vi "Open Section Datas.vi"(8 "error in (no error)":errorcluster, 11 "Data in":string) -> (0 "error out":errorcluster, 3 "Section":refnum<data-value>)   [LabVIEW 2013, in "Hierarchy Framework.lvlib" / "Section.lvclass"]
uses:
  Section.lvclass
  Channel/Channel.lvclass
  Channel/Ctls/Dimensions.ctl
  Item/Item.lvclass
  Generic/Generic.lvclass
panel:
  out "String":string
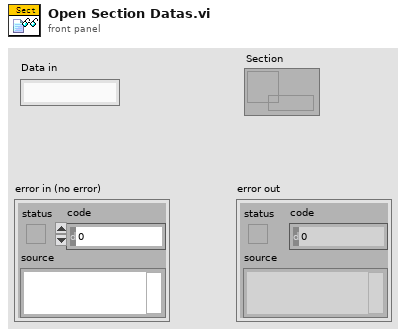
[diagram p1: front panel]
types:
  T1 = typedef "Hierarchy Framework.lvlib/Channel.lvclass/Dimensions.ctl" = cluster{"Row":i32, "Column":i32}
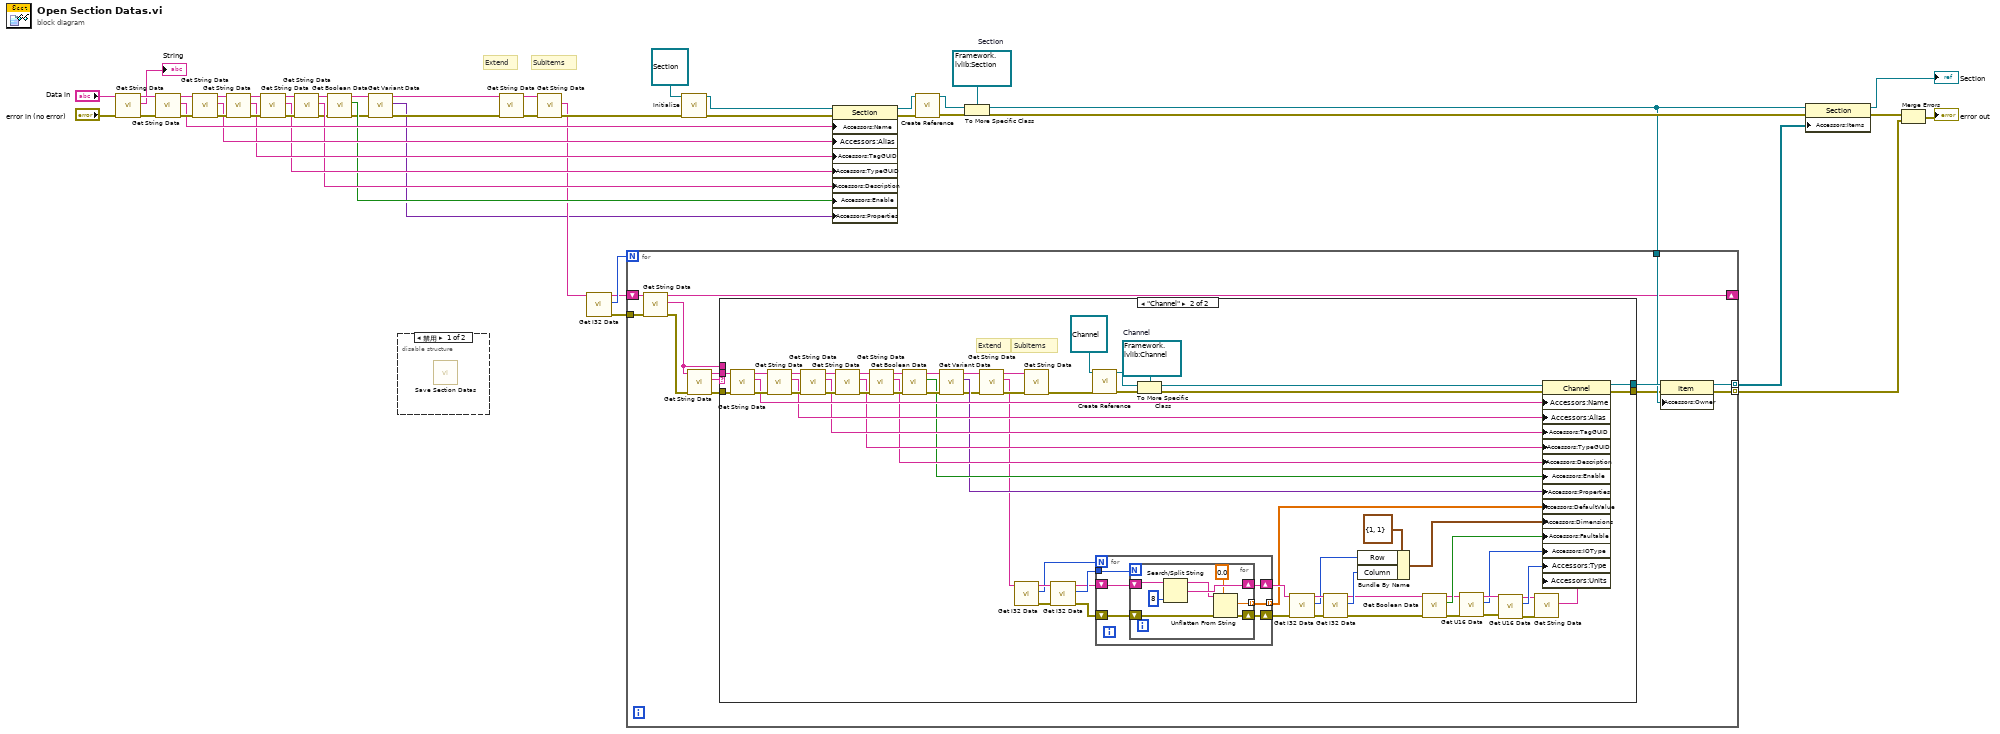
[diagram p0: block diagram]
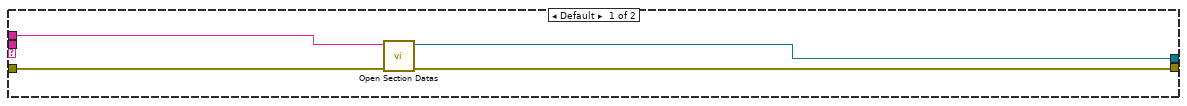
[diagram p2: hidden frame]
diagram:
  w45 = refnum<data-value> refnum  # Section
  # "SubItems"
  # "Extend"
  n1 = call "Get String Data.vi"("error in (no error)"="error in (no error)", "Data in"="Data in") -> ("error out"=w33:errorcluster, "String"=→"String":string, "Data out"=w34:string)  [unwired: 7 in]
  n2 = call "Get String Data.vi"("error in (no error)"=w33, "Data in"=w34) -> ("error out"=w26:errorcluster, "String"=w24:string, "Data out"=w28:string)  [unwired: 7 in]
  n3 = call "Get String Data.vi"("error in (no error)"=w26, "Data in"=w28) -> ("error out"=w32:errorcluster, "String"=w23:string, "Data out"=w31:string)  [unwired: 7 in]
  n4 = call "Get String Data.vi"("error in (no error)"=w32, "Data in"=w31) -> ("error out"=w25:errorcluster, "String"=w22:string, "Data out"=w27:string)  [unwired: 7 in]
  n5 = call "Get String Data.vi"("error in (no error)"=w25, "Data in"=w27) -> ("error out"=w29:errorcluster, "String"=w21:string, "Data out"=w30:string)  [unwired: 7 in]
  n6 = call "Get String Data.vi"("error in (no error)"=w29, "Data in"=w30) -> ("error out"=w17:errorcluster, "String"=w20:string, "Data out"=w18:string)  [unwired: 7 in]
  n7 = call "Get Boolean Data.vi"("error in (no error)"=w17, "Data in"=w18) -> ("error out"=w7:errorcluster, "Boolean"=w16:bool, "Data out"=w8:string)  [unwired: 7 in]
  n8 = call "Get Variant Data.vi"("error in (no error)"=w7, "Data in"=w8) -> ("error out"=w5:errorcluster, "Variant"=w4:variant, "Data out"=w6:string)  [unwired: 7 in]
  n9 = disable-structure shown="禁用" {
    frame Disabled {
      n10 = call "Save Section Datas.vi"() -> ()  [unwired: 9 in, 3 out]
    }
    frame Enabled {
    }
  }
  n11 = call "Get String Data.vi"("error in (no error)"=w5, "Data in"=w6) -> ("error out"=w15:errorcluster, "Data out"=w14:string)  [unwired: 7 in, 1 out]
  n12 = call "Get String Data.vi"("error in (no error)"=w15, "Data in"=w14) -> ("error out"=w13:errorcluster, "String"=w9:string)  [unwired: 7 in, 1 out]
  n13 = call "Get I32 Data.vi"("Data in"=w9) -> ("error out"=w10:errorcluster, "I32"=w12:i32, "Data out"=w11:string)  [unwired: 8 in]
  n14 = call-dynamic "Initialize.vi"("error in (no error)"=w13, "Section输入"=refnum<class "Section.lvclass"> refnum ("Framework.lvlib:Section")) -> ("error out"=w39:errorcluster, "Section输出"=w38:refnum<class "Section.lvclass">)  [unwired: 8 in]
  n15 = property class="Section"(reference=w38, error in=w39, "Accessors:Name"=w24, "Accessors:Alias"=w23, "Accessors:TagGUID"=w22, "Accessors:TypeGUID"=w21, "Accessors:Description"=w20, "Accessors:Enable"=w16, "Accessors:Properties"=w4) -> (reference out=w41:refnum<class "Section.lvclass">, error out=w42:errorcluster)
  n16 = call "Create Reference.vi"("error in (no error)"=w42, "Generic"=w41) -> ("error out"=w44:errorcluster, "Generic Reference"=w43:refnum<data-value>)  [unwired: 8 in]
  n17 = To More Specific Class(target class=w45, reference=w43, error in=w44) -> (specific class reference=w37:refnum<data-value>, error out=w46:errorcluster)
  n18 = for {
    N: w12 -> [_]
    tunnel: [w60] -> w47 mode=indexing
    tunnel: w37 -> [w59]
    shift-right: [w57] -> _
    shift-left: w11 -> [w58]
    tunnel: w10 -> [w56]
    tunnel: [w49] -> w2 mode=indexing
    n19 = call "Get String Data.vi"("error in (no error)"=w56, "Data in"=w58) -> ("error out"=w51:errorcluster, "String"=w52:string, "Data out"=w57:string)  [unwired: 7 in]
    n20 = call "Get String Data.vi"("error in (no error)"=w51, "Data in"=w52) -> ("error out"=w53:errorcluster, "String"=w55:string, "Data out"=w54:string)  [unwired: 7 in]
    n21 = case shown="\"Channel\"" w55 {
      tunnel: [w65 w121] -> w61
      tunnel: w54 -> [_ w112]
      tunnel: w53 -> [w63 w111]
      tunnel: w52 -> [w64 _]
      tunnel: [w62 w66] -> w50
      frame Default {
        n22 = call "Open Section Datas.vi"("error in (no error)"=w63, "Data in"=w64) -> ("error out"=w62:errorcluster, "Section"=w65:refnum<data-value>)  [unwired: 8 in]
      }
      frame "Channel" {
        w124 = refnum<data-value> refnum  # Channel
        # "SubItems"
        # "Extend"
        n23 = call "Get String Data.vi"("error in (no error)"=w111, "Data in"=w112) -> ("error out"=w110:errorcluster, "String"=w104:string, "Data out"=w118:string)  [unwired: 7 in]
        n24 = call "Get String Data.vi"("error in (no error)"=w110, "Data in"=w118) -> ("error out"=w109:errorcluster, "String"=w103:string, "Data out"=w120:string)  [unwired: 7 in]
        n25 = call "Get String Data.vi"("error in (no error)"=w109, "Data in"=w120) -> ("error out"=w108:errorcluster, "String"=w102:string, "Data out"=w117:string)  [unwired: 7 in]
        n26 = call "Get String Data.vi"("error in (no error)"=w108, "Data in"=w117) -> ("error out"=w107:errorcluster, "String"=w101:string, "Data out"=w119:string)  [unwired: 7 in]
        n27 = call "Get String Data.vi"("error in (no error)"=w107, "Data in"=w119) -> ("error out"=w106:errorcluster, "String"=w100:string, "Data out"=w116:string)  [unwired: 7 in]
        n28 = call "Get Boolean Data.vi"("error in (no error)"=w106, "Data in"=w116) -> ("error out"=w105:errorcluster, "Boolean"=w99:bool, "Data out"=w115:string)  [unwired: 7 in]
        n29 = call "Get Variant Data.vi"("error in (no error)"=w105, "Data in"=w115) -> ("error out"=w67:errorcluster, "Variant"=w98:variant, "Data out"=w114:string)  [unwired: 7 in]
        n30 = call "Get String Data.vi"("error in (no error)"=w67, "Data in"=w114) -> ("error out"=w97:errorcluster, "String"=w95:string, "Data out"=w113:string)  [unwired: 7 in]
        n31 = call "Get I32 Data.vi"("Data in"=w95) -> ("error out"=w93:errorcluster, "I32"=w92:i32, "Data out"=w94:string)  [unwired: 8 in]
        n32 = call "Get String Data.vi"("error in (no error)"=w97, "Data in"=w113) -> ("error out"=w96:errorcluster)  [unwired: 7 in, 2 out]
        n33 = call "Get I32 Data.vi"("error in (no error)"=w93, "Data in"=w94) -> ("error out"=w89:errorcluster, "I32"=w91:i32, "Data out"=w90:string)  [unwired: 7 in]
        n34 = call "Create Reference.vi"("error in (no error)"=w96, "Generic"=refnum<class "Channel.lvclass"> refnum ("Framework.lvlib:Channel")) -> ("error out"=w125:errorcluster, "Generic Reference"=w126:refnum<data-value>)  [unwired: 8 in]
        n35 = for {
          N: w92 -> [_]
          shift-right: [w131] -> w86
          shift-left: w90 -> [w132]
          tunnel: w91 -> [w133]
          tunnel: [w130] -> w85 mode=indexing
          shift-right: [w128] -> w84
          shift-left: w89 -> [w129]
          n36 = for {
            N: w133 -> [_]
            shift-right: [w139] -> w131
            shift-left: w132 -> [w141]
            tunnel: [w136] -> w130 mode=indexing
            shift-right: [w134] -> w128
            shift-left: w129 -> [w135]
            n37 = Search/Split String(string=w141, offset (0)=8 ("偏移量(0)")) -> (substring before match=w138:string, match + rest of string=w139:string)  [unwired: 1 in, 1 out]
            n38 = Unflatten From String(type=0.0 ("数值"), binary string=w138, error in (no error)=w135) -> (value=w136:dbl, error out=w134:errorcluster)  [unwired: 2 in, 1 out]
          }
        }
        n39 = To More Specific Class(target class=w124, reference=w126, error in=w125) -> (specific class reference=w123:refnum<data-value>, error out=w122:errorcluster)
        n40 = call "Get I32 Data.vi"("error in (no error)"=w84, "Data in"=w86) -> ("error out"=w88:errorcluster, "I32"=w81:i32, "Data out"=w87:string)  [unwired: 7 in]
        n41 = call "Get I32 Data.vi"("error in (no error)"=w88, "Data in"=w87) -> ("error out"=w78:errorcluster, "I32"=w80:i32, "Data out"=w79:string)  [unwired: 7 in]
        n42 = Bundle By Name(cluster=T1 {"Row"=1, "Column"=1} ("Dimensions"), "Row"=w81, "Column"=w80) -> (w82:T1)
        n43 = call "Get Boolean Data.vi"("error in (no error)"=w78, "Data in"=w79) -> ("error out"=w73:errorcluster, "Boolean"=w77:bool, "Data out"=w74:string)  [unwired: 7 in]
        n44 = call "Get U16 Data.vi"("error in (no error)"=w73, "Data in"=w74) -> ("error out"=w76:errorcluster, "U16"=w72:u16, "Data out"=w75:string)  [unwired: 7 in]
        n45 = call "Get U16 Data.vi"("error in (no error)"=w76, "Data in"=w75) -> ("error out"=w70:errorcluster, "U16"=w71:u16, "Data out"=w69:string)  [unwired: 7 in]
        n46 = call "Get String Data.vi"("error in (no error)"=w70, "Data in"=w69) -> ("String"=w68:string)  [unwired: 7 in, 2 out]
        n47 = property class="Channel"(reference=w123, error in=w122, "Accessors:Name"=w104, "Accessors:Alias"=w103, "Accessors:TagGUID"=w102, "Accessors:TypeGUID"=w101, "Accessors:Description"=w100, "Accessors:Enable"=w99, "Accessors:Properties"=w98, "Accessors:DefaultValue"=w85, "Accessors:Dimensions"=w82, "Accessors:Faultable"=w77, "Accessors:IOType"=w72, "Accessors:Type"=w71, "Accessors:Units"=w68) -> (reference out=w121:refnum<data-value>, error out=w66:errorcluster)
      }
    }
    n48 = property class="Item"(reference=w61, error in=w50, "Accessors:Owner"=w59) -> (reference out=w60:refnum<data-value>, error out=w49:errorcluster)
  }
  n49 = property class="Section"(reference=w37, error in=w46, "Accessors:Items"=w47) -> (reference out=→"Section":refnum<data-value>, error out=w3:errorcluster)
  n50 = Merge Errors(w3, w2) -> (→"error out":errorcluster)
